vi "Handle Error.vi"(8 "error in (no error)":errorcluster, 11 "OOQMH in":refnum<class "OOQMH.lvclass">) -> (0 "error out":errorcluster, 3 "OOQMH out":refnum<class "OOQMH.lvclass">, 4 "stop?":bool)   [LabVIEW 2024, in "OOQMH.lvlib" / "OOQMH.lvclass"]
uses:
  OOQMH.lvclass
  OOQMH.lvclass/OOQMH.ctl
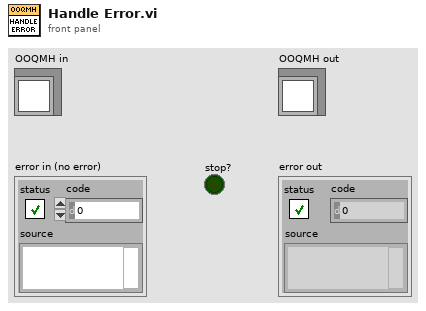
[diagram p1: front panel]
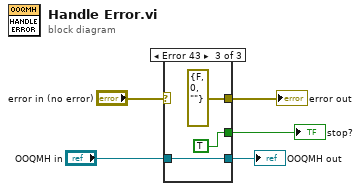
[diagram p0: block diagram]
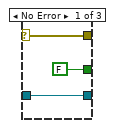
[diagram p2: hidden frame]
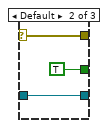
[diagram p3: hidden frame]
diagram:
  n1 = case shown="Error 43" "error in (no error)" {
    selector: "error in (no error)" -> [w7 w11 _]
    tunnel: [w7 w11 errorcluster {"status"=FALSE, "code"=0, "source"=""} ("error constant")] -> w4
    tunnel: [w8 w10 w14] -> w2
    tunnel: "OOQMH in" -> [w8 w10 w14]
    tunnel: [FALSE TRUE TRUE] -> w1
    frame No Error {
    }
    frame Default {
    }
    frame Error {
    }
  }
  "error out" <- w4
  "OOQMH out" <- w2
  "stop?" <- w1
